vi "Get App Version.vi"() -> (0 "App. Version Number":string, 1 "runtime":bool)   [LabVIEW 2013]
doc: "Returns application version number for compiled exe file. In the case of developement or other, returns describing text."
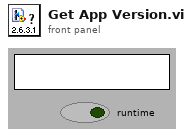
[diagram p1: front panel]
types:
  T1 = enum32{"invalid app kind", "Development System", "Run Time System", "Student Edition", "Embedded LabVIEW", "Evaluation", "Custom"}
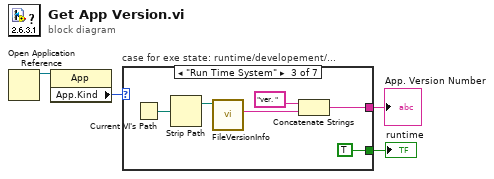
[diagram p0: block diagram]
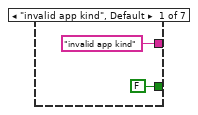
[diagram p2: hidden frame]
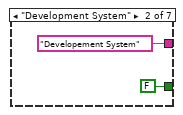
[diagram p3: hidden frame]
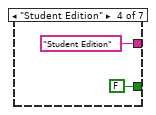
[diagram p4: hidden frame]
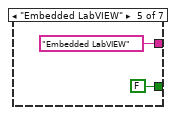
[diagram p5: hidden frame]
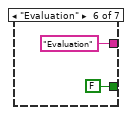
[diagram p6: hidden frame]
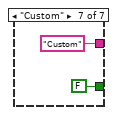
[diagram p7: hidden frame]
diagram:
  n1 = Open Application Reference() -> (3:w4:refnum<vi>)  [unwired: 4 in, 1 out]
  n2 = property class="App"(reference=w4) -> ("App.Kind"=w3:T1)  [unwired: 1 in, 2 out]
  n3 = case "case for exe state: runtime/developement/..." shown="\"Run Time System\"" w3 {
    tunnel: ["invalid app kind" "Developement System" w10 "Student Edition" "Embedded LabVIEW" "Evaluation" "Custom"] -> w2
    tunnel: [FALSE ("runtime") FALSE ("runtime") TRUE ("runtime") FALSE ("runtime") FALSE ("runtime") FALSE ("runtime") FALSE ("runtime")] -> w1
    frame "invalid app kind", Default {
    }
    frame "Development System" {
    }
    frame "Run Time System" {
      n4 = Current VI's Path() -> (path=w11:path)
      n5 = Strip Path(path=w11) -> (stripped path=w12:path)  [unwired: 1 out]
      n6 = call <vilib>:"FileVersionInfo.vi"("Application Path in"=w12) -> ("File Version Info"=w13:string)  [unwired: 7 in, 3 out]
      n7 = Concatenate Strings("ver. " ("string"), w13) -> (w10:string)
    }
    frame "Student Edition" {
    }
    frame "Embedded LabVIEW" {
    }
    frame "Evaluation" {
    }
    frame "Custom" {
    }
  }
  "App. Version Number" <- w2
  "runtime" <- w1
